vi "WPI_CameraIssue Get.vi"(7 "address":string, 8 "error in (no error)":errorcluster, 9 "Regular Expression of text to extract":string=".*", 10 "Number of Lines Expected":i32=1, 11 "Request":string) -> (0 "error out":errorcluster, 1 "Complete Response":string, 2 "offset past match":i32, 3 "Extracted String":string)   [LabVIEW 2017]
doc: "Issues a GET TCP request. Checks whether the request was succesful. If success, then matches the given regular expression against the response and returns the matched portion.\n\nThis software is licensed. Open the labview\\readme\\WPI Robotics Library Open Source License.txt file for more information."
panel:
  out "Camera Request":string
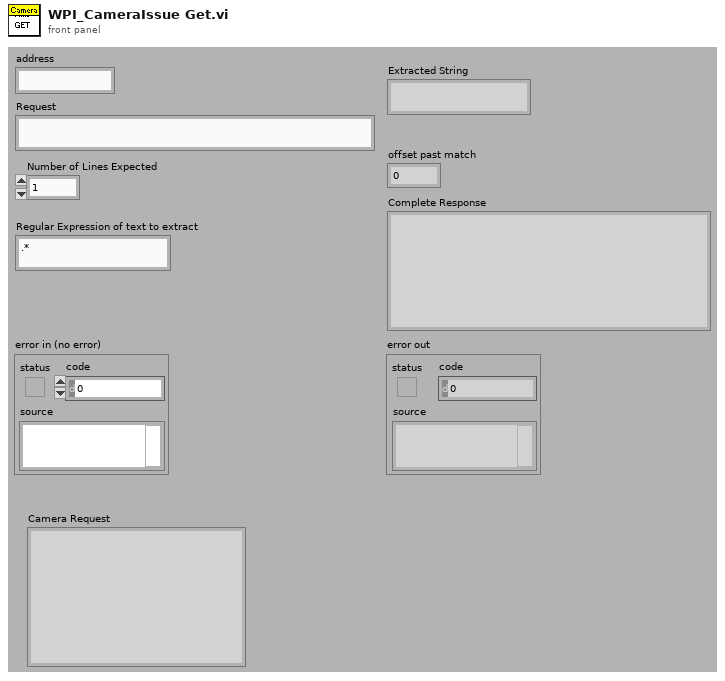
[diagram p1: front panel]
types:
  T1 = enum16{"Standard", "Buffered", "CRLF", "Immediate"}
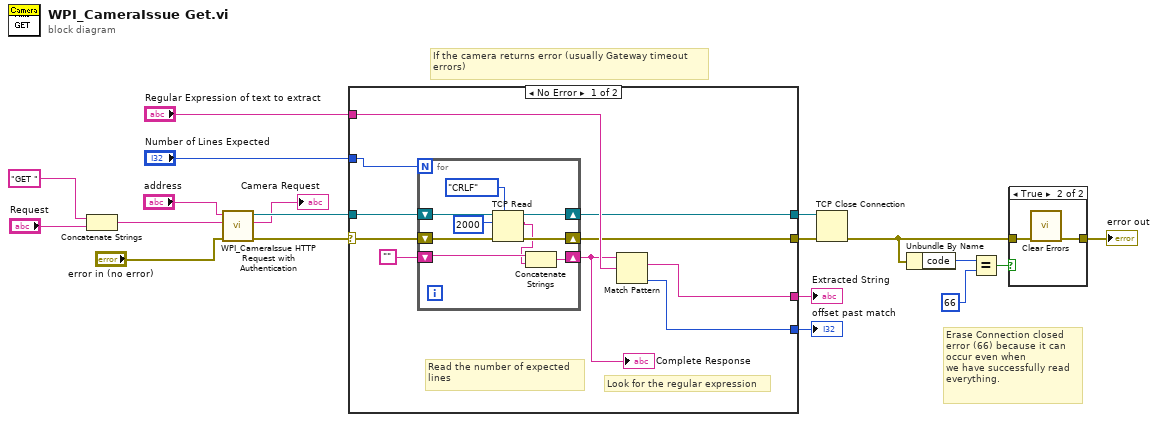
[diagram p0: block diagram]
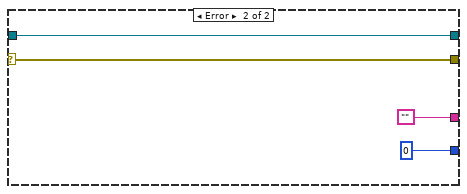
[diagram p3: hidden frame]
diagram:
  # "Erase Connection closed\nerror (66) because it can\noccur even when \nwe have successfully read\neverything."
  # "If the camera returns error (usually Gateway timeout\nerrors)"
  n1 = Concatenate Strings("GET " ("string"), "Request") -> (w15:string)
  n2 = call <vilib>:"WPI_CameraIssue HTTP Request with Authentication.vi"("error in (no error)"="error in (no error)", "Request"=w15, "address"="address") -> ("error out"=w9:errorcluster, "Authenticated request"=→"Camera Request":string, "connection ID (dup)"=w10:refnum<k5>)  [unwired: 2 in, 4 out]
  n3 = case shown="No Error" w9 {
    selector: w9 -> [w20 w39]
    tunnel: "Regular Expression of text to extract" -> [w29 _]
    tunnel: [w28 0 ("offset past match")] -> w18
    tunnel: "Number of Lines Expected" -> [w21 _]
    tunnel: w10 -> [w25 w42]
    tunnel: [w24 w42] -> w12
    tunnel: [w23 ""] -> w16
    tunnel: [w22 w39] -> w11
    frame No Error {
      # "Look for the regular expression"
      # "Read the number of expected\nlines"
      n4 = for {
        N: w21 -> [_]
        shift-right: [w30] -> w27
        shift-left: "" -> [w32]
        shift-right: [w34] -> w24
        shift-left: w25 -> [w36]
        shift-right: [w33] -> w22
        shift-left: w20 -> [w35]
        n5 = TCP Read(connection ID=w36, bytes to read=2000, error in (no error)=w35, 7:T1."CRLF" ("mode (standard)")) -> (connection ID out=w34:refnum<k5>, data out=w31:string, error out=w33:errorcluster)  [unwired: 1 out]
        n6 = Concatenate Strings(w32, w31) -> (w30:string)
      }
      "Complete Response" <- w27
      n7 = Match Pattern(string=w27, regular expression=w29) -> (match substring=w23:string, offset past match=w28:i32)  [unwired: 1 in, 2 out]
    }
    frame Error {
    }
  }
  "offset past match" <- w18
  "Extracted String" <- w16
  n8 = TCP Close Connection(connection ID=w12, error in (no error)=w11) -> (error out=w3:errorcluster)  [unwired: 2 out]
  n9 = Unbundle By Name(w3) -> ("code"=w6:i32)
  n10 = Equal?(x=w6, y=66) -> (x = y?=w4:bool)
  n11 = case shown="True" w4 {
    tunnel: w3 -> [w43 w45]
    tunnel: [w43 w44] -> w1
    frame False {
    }
    frame True {
      n12 = call <vilib>:"Clear Errors.vi"("error in (no error)"=w45) -> ("error out"=w44:errorcluster)  [unwired: 1 in, 5 out]
    }
  }
  "error out" <- w1
